vi "receiveSerialNumber.vi"(8 "error in (no error)":errorcluster, 11 "ILC in":refnum<class "ILC.lvclass">) -> (0 "error out":errorcluster, 2 "Serial Number":string, 3 "ILC out":refnum<class "ILC.lvclass">)   [LabVIEW 2015, in "ILCCommon.lvlib" / "ILC.lvclass"]
uses:
  <userlib>/Common/ILC/ILC/ILC.lvclass
  <userlib>/Common/SerialProtocols/SerialCommunicator/SerialCommunicator.lvclass
  <userlib>/Common/ILC/ILCModelTypedefs/FinalDelimiter.ctl
  <userlib>/Common/ILC/ILCModelTypedefs/ILCModelTypedefs.lvlib
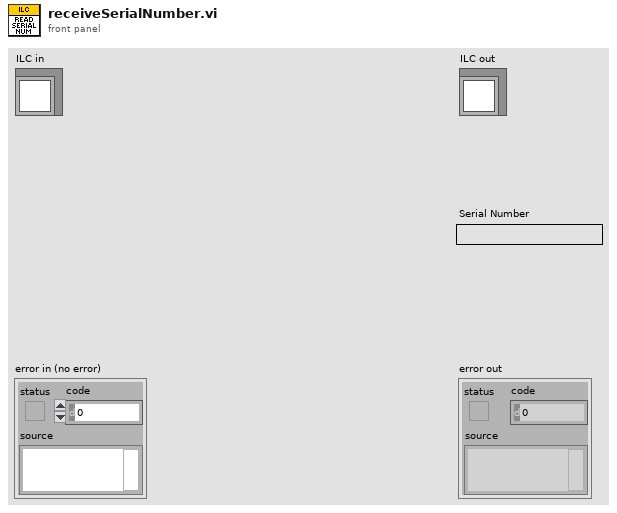
[diagram p1: front panel]
types:
  T1 = typedef "ILCCommon.lvlib/ILCModelTypedefs.lvlib/FinalDelimiter.ctl" = enum16{",", "<CR><LF>"}
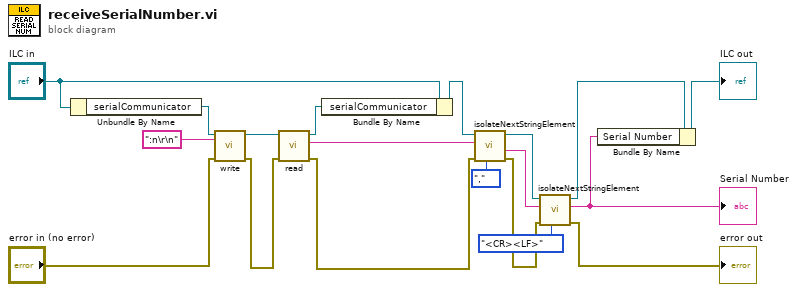
[diagram p0: block diagram]
diagram:
  n1 = Unbundle By Name("ILC in") -> ("serialCommunicator"=w12:refnum<class "SerialCommunicator.lvclass">)
  n2 = call-dynamic "write.vi"("error in (no error)"="error in (no error)", "writeString"=":n\r\n", "SerialCommunicator in"=w12) -> ("error out"=w7:errorcluster, "SerialCommunicator out"=w14:refnum<class "SerialCommunicator.lvclass">)  [unwired: 7 in]
  n3 = call-dynamic "read.vi"("error in (no error)"=w7, "SerialCommunicator in"=w14) -> ("error out"=w4:errorcluster, "stringRead"=w15:string, "SerialCommunicator out"=w5:refnum<class "SerialCommunicator.lvclass">)  [unwired: 7 in]
  n4 = Bundle By Name(cluster="ILC in", "serialCommunicator"=w5) -> (w2:refnum<class "ILC.lvclass">)
  n5 = call <userlib>:"isolateNextStringElement.vi"("Final Delimiter"=FinalDelimiter.",", "error in (no error)"=w4, "inputString"=w15, "ILC in"=w2) -> ("error out"=w3:errorcluster, "remainingString"=w17:string, "ILC out"=w16:refnum<class "ILC.lvclass">)  [unwired: 4 in, 1 out]
  n6 = call <userlib>:"isolateNextStringElement.vi"("Final Delimiter"=FinalDelimiter."<CR><LF>", "error in (no error)"=w3, "inputString"=w17, "ILC in"=w16) -> ("error out"=→"error out":errorcluster, "extractedSegment"=w9:string, "ILC out"=w1:refnum<class "ILC.lvclass">)  [unwired: 4 in, 1 out]
  "Serial Number" <- w9
  n7 = Bundle By Name(cluster=w1, "Serial Number"=w9) -> (→"ILC out":refnum<class "ILC.lvclass">)
